vi "Main.vi"() -> ()   [LabVIEW 2020]
doc: "Use this template to build a simple state machine design pattern. Each state executes code and determines which state to transition to."
uses:
  controls/State.ctl
  controls/Data.ctl
  <vilib>/DAQmx/configure/timing.llb/DAQmx Timing (Sample Clock).vi
  <vilib>/DAQmx/create/channels.llb/DAQmx Create Channel (AI-Voltage-Basic).vi
  <vilib>/daqmxs/DAQmx sim.lvlib
  <vilib>/Waveform/WDTOps.llb/WDT Append Waveforms DBL.vi
  <vilib>/daqmxs/DAQmx Read sim (Analog Wfm 1Chan NSamp).vi
panel:
  in  "git pokus":bool
  in  "Init measurement":bool
  in  "stop":bool
  out "Waveform Graph":waveform(dbl)(graph)
  in  "Start Measurement":bool
  in  "rate":dbl=1000.0
  in  "physical channels 2":tag
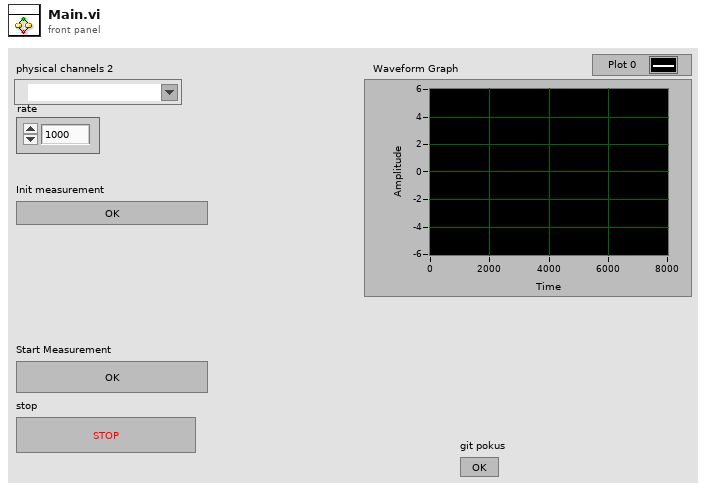
[diagram p1: front panel]
types:
  T1 = typedef "Data.ctl" = cluster{"Boolean ":bool, "String <Replace Me>":string, "Numeric <Replace Me>":dbl, "task out":refnum<k21>, "Waveform":waveform(dbl), "Numeric":i32}
  T2 = typedef "State.ctl" = enum16{"Initialize", "Wait for Event", "Run_measurement", "Exit", "Stop_measurement", "Read_measurement", "Init_measurement"}
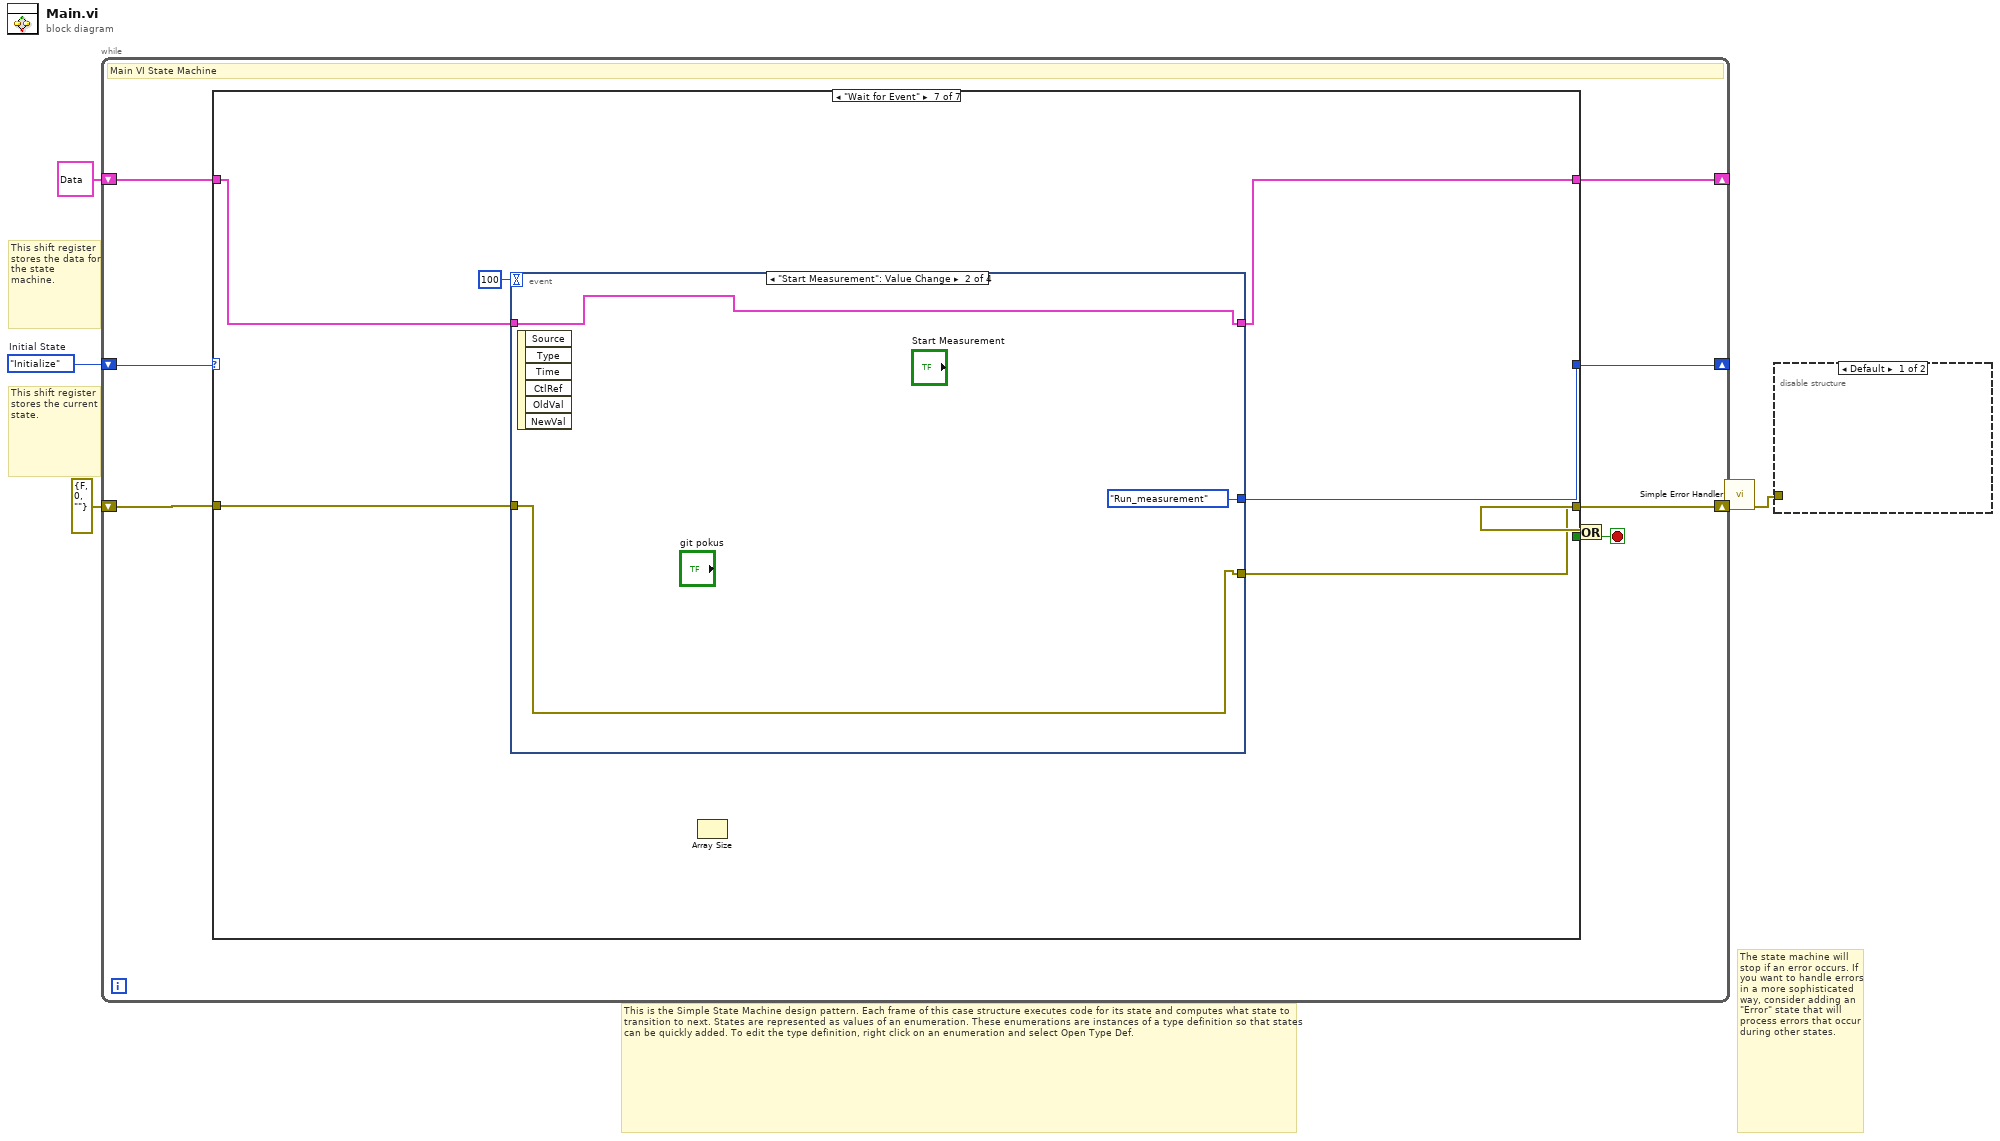
[diagram p0: block diagram]
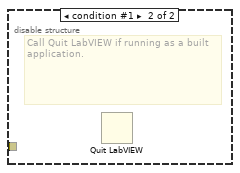
[diagram p2: hidden frame]
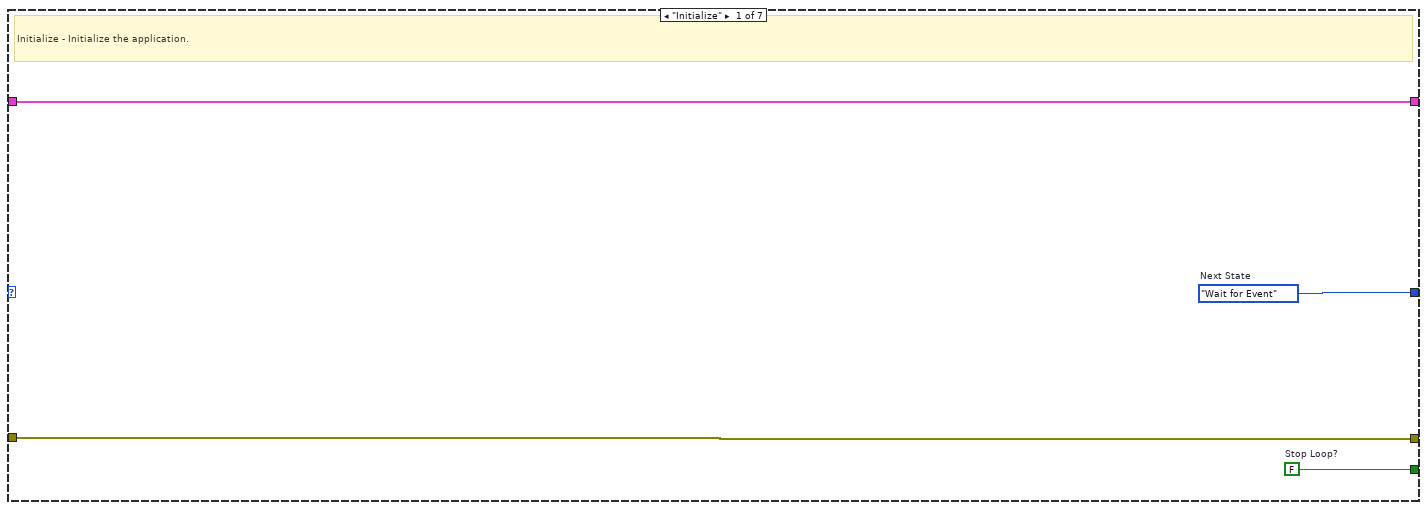
[diagram p3: hidden frame]
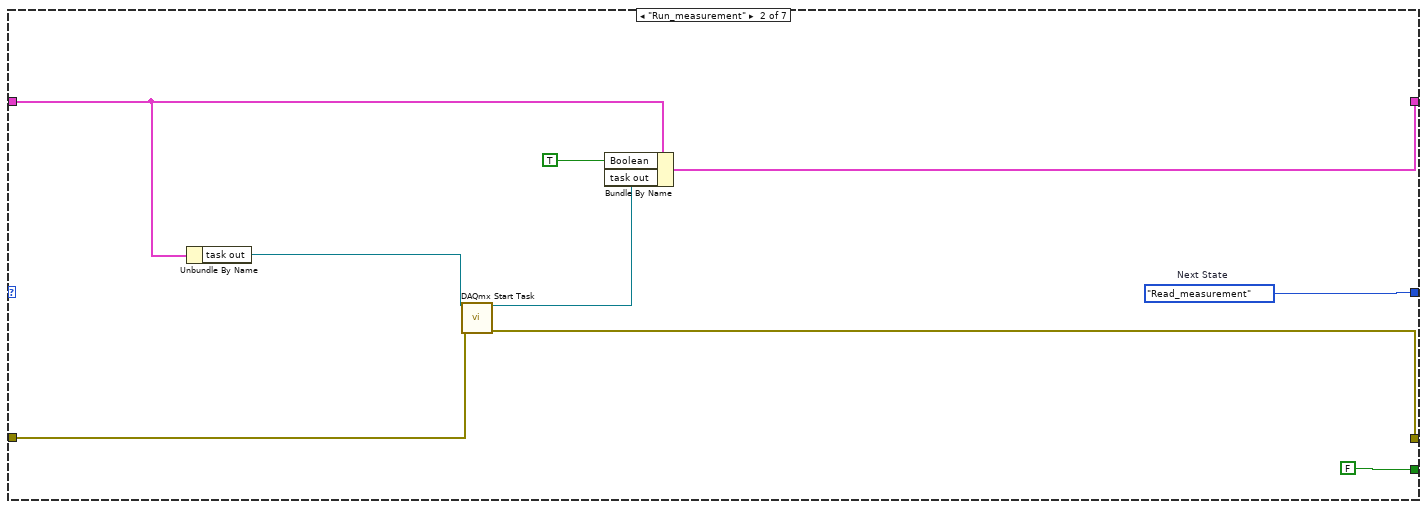
[diagram p4: hidden frame]
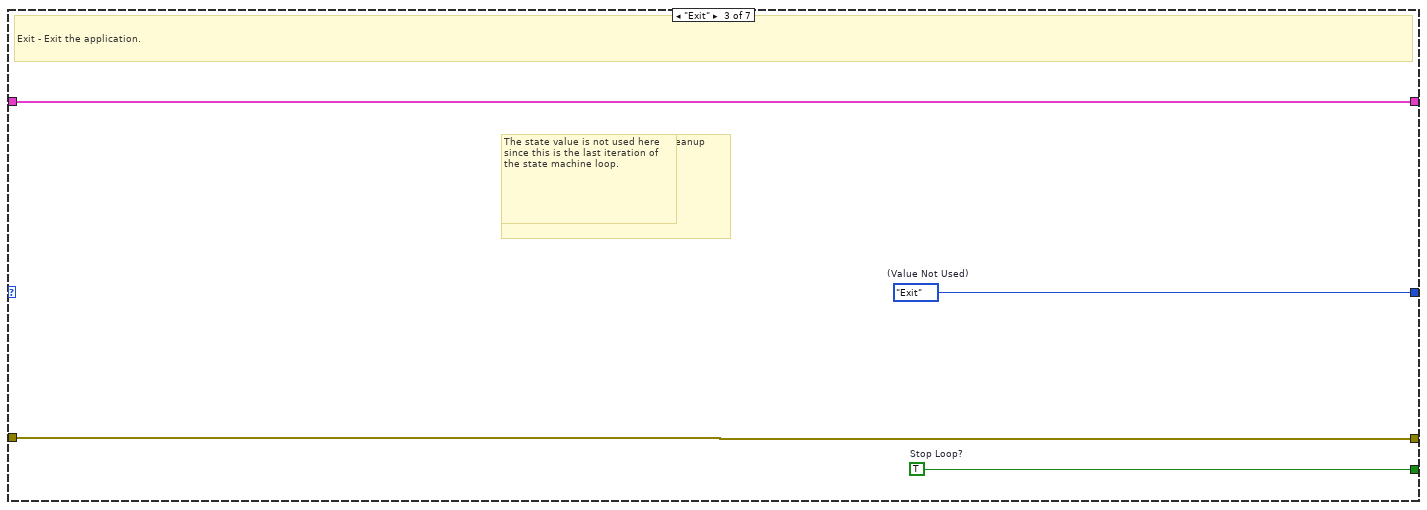
[diagram p5: hidden frame]
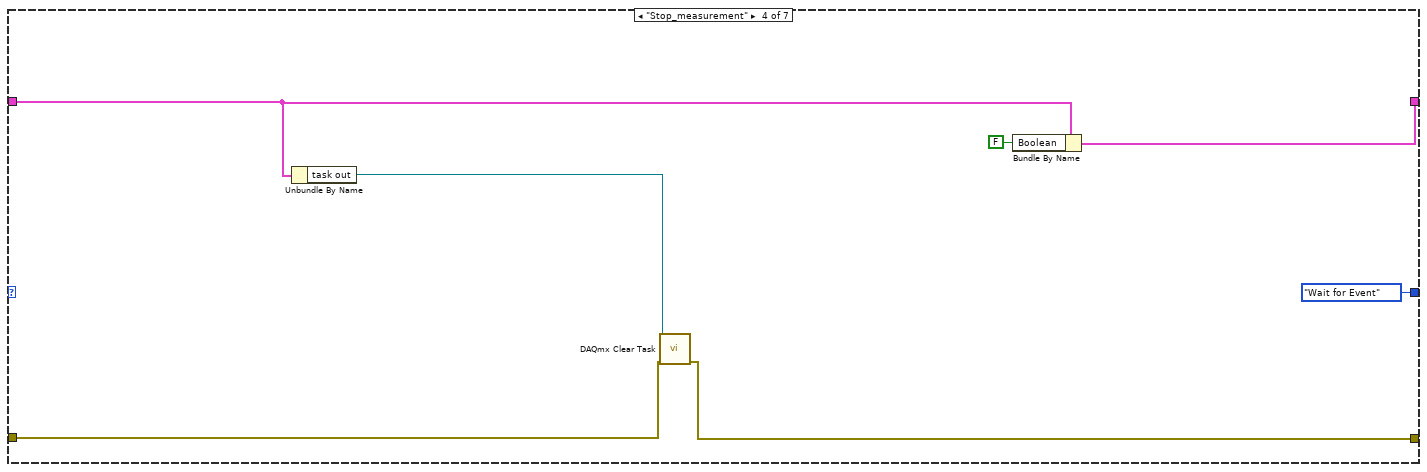
[diagram p6: hidden frame]
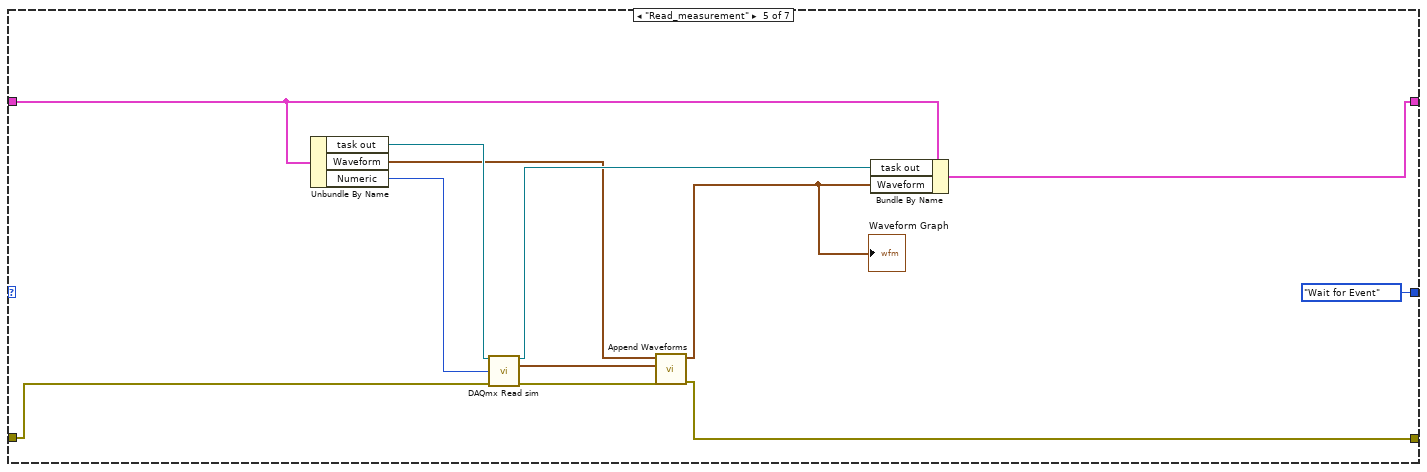
[diagram p7: hidden frame]
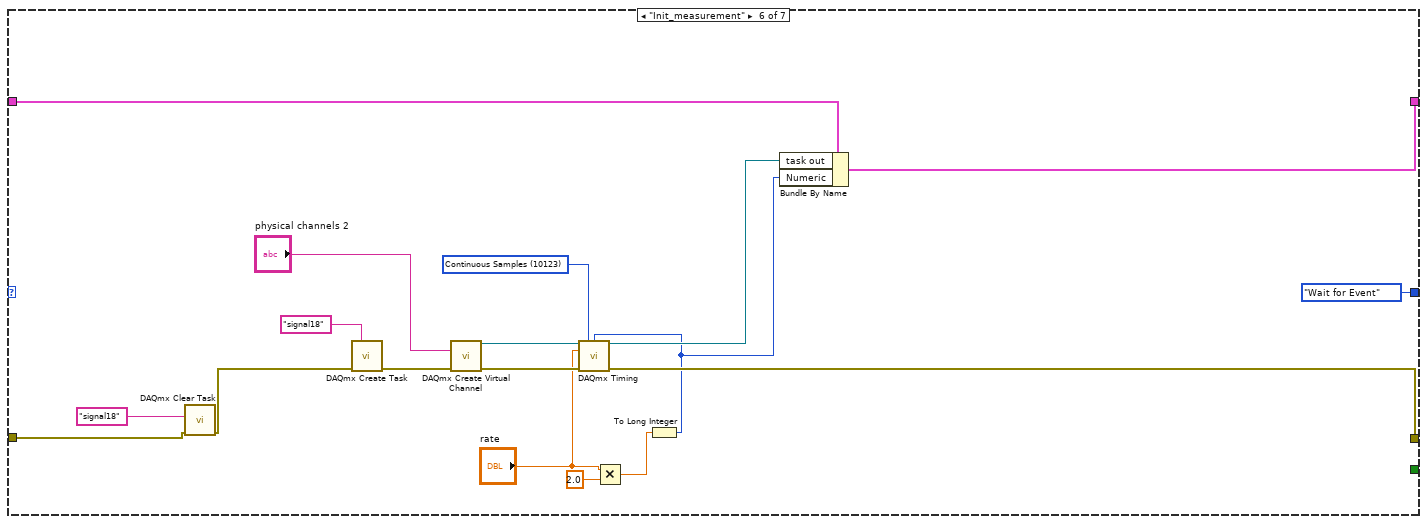
[diagram p8: hidden frame]
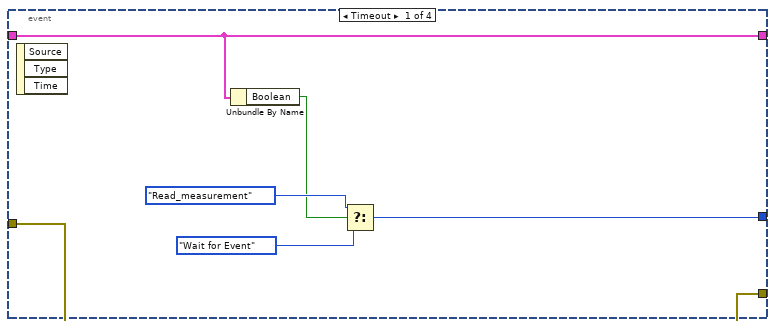
[diagram p9: hidden frame]
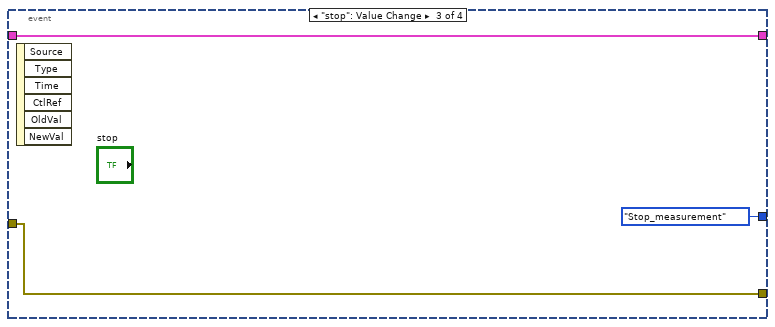
[diagram p10: hidden frame]
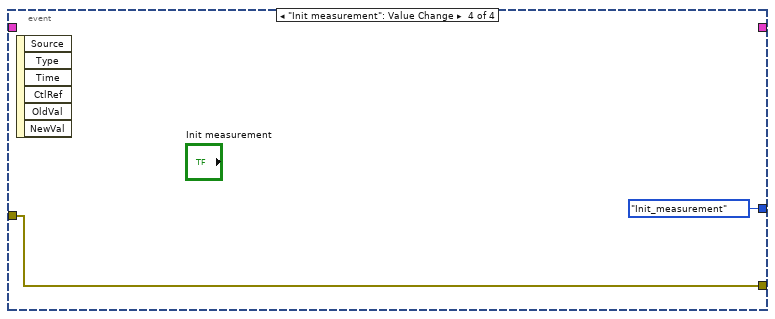
[diagram p11: hidden frame]
diagram:
  w5 = State."Initialize"  # Initial State
  # "The state machine will stop if an error occurs. If you want to handle errors in a more sophisticated way, consider adding an \"Error\" state that will process errors that occur during other states."
  # "This shift register stores the data for the state machine."
  # "This is the Simple State Machine design pattern. Each frame of this case structure executes code for its state and computes what state to transition to next. States are represented as values of an enumeration. These enumerations are instances of a type definition so that states can be quickly added. To edit the type definition, right click on an enumeration and select Open Type Def."
  # "This shift register stores the current state."
  n1 = while {
    shift-right: [w12] -> _
    shift-left: w5 -> [w13]
    shift-right: [w10] -> _
    shift-left: T1 {"Boolean "=FALSE, "String <Replace Me>"="", "Numeric <Replace Me>"=0.0, "task out"="", "Waveform"={"t0"=timestamp(0 s since 1904-01-01), "dt"=1.0, "Y"=[]}, "Numeric"=0} ("Data") -> [w11]
    shift-right: [w6] -> w2
    shift-left: errorcluster {"status"=FALSE, "code"=0, "source"=""} ("error constant") -> [w9]
    stop <- w7 stop-if-true
    # "Main VI State Machine"
    n2 = case shown="\"Wait for Event\"" w13 {
      tunnel: [w17 w25 w30 State."Wait for Event" ("(Value Not Used)") State."Wait for Event" ("(Value Not Used)") State."Wait for Event" ("(Value Not Used)") w72] -> w12
      tunnel: [w16 FALSE ("Stop Loop?") w28 _ _ _ _] -> w8
      tunnel: w11 -> [w14 w21 w29 w34 w47 w58 w69]
      tunnel: [w14 w20 w29 w33 w46 w57 w68] -> w10
      tunnel: w9 -> [w15 w24 w27 w36 w40 w59 w71]
      tunnel: [w15 w23 w27 w35 w39 w54 w70] -> w6
      frame "Initialize" {
        w16 = FALSE  # Stop Loop?
        w17 = State."Wait for Event"  # Next State
        # "Initialize - Initialize the application."
      }
      frame "Run_measurement" {
        w25 = State."Read_measurement"  # Next State
        n3 = Unbundle By Name(w21) -> ("task out"=w22:refnum<k21>)
        n4 = call <vilib>:"DAQmx Start Task.vi"("task/channels in"=w22, "error in"=w24) -> ("task out"=w19:refnum<k21>, "error out"=w23:errorcluster)  [unwired: 12 in]
        n5 = Bundle By Name(cluster=w21, "Boolean"=TRUE ("Boolean <Replace Me>"), "task out"=w19) -> (w20:T1)
      }
      frame "Exit" {
        w28 = TRUE  # Stop Loop?
        w30 = State."Exit"  # (Value Not Used)
        # "#CodeNeeded - Add any required cleanup code here."
        # "The state value is not used here since this is the last iteration of the state machine loop."
        # "Exit - Exit the application."
      }
      frame "Stop_measurement" {
        n6 = Unbundle By Name(w34) -> ("task out"=w37:refnum<k21>)
        n7 = call <vilib>:"DAQmx Clear Task.vi"("task in"=w37, "error in"=w36) -> ("error out"=w35:errorcluster)  [unwired: 13 in]
        n8 = Bundle By Name(cluster=w34, "Boolean"=FALSE) -> (w33:T1)
      }
      frame "Read_measurement" {
        n9 = Unbundle By Name(w47) -> ("task out"=w48:refnum<k21>, "Waveform"=w44:waveform(dbl), "Numeric"=w38:i32)
        n10 = call-poly <vilib>:"DAQmx Read sim.vi"("task/channels in"=w48, "number of samples per channel"=w38, "error in"=w40) -> ("task out"=w45:refnum<k21>, "data"=w43:waveform(dbl), "error out"=w41:errorcluster)  [unwired: 10 in]
        n11 = call-poly <vilib>:"Append Waveforms.vi"("error in (no error)"=w41, "waveform B"=w43, "waveform A"=w44) -> ("error out"=w39:errorcluster, "waveform out"=w42:waveform(dbl))  [unwired: 7 in]
        "Waveform Graph" <- w42
        n12 = Bundle By Name(cluster=w47, "task out"=w45, "Waveform"=w42) -> (w46:T1)
      }
      frame "Init_measurement" {
        w61 = 10123 items=["Finite Samples"=10178, "Continuous Samples"=10123, "Hardware Timed Single Point"=12522] ("sample mode")
        n13 = call <vilib>:"DAQmx Clear Task.vi"("task in"="signal18" ("new task name"), "error in"=w59) -> ("error out"=w60:errorcluster)  [unwired: 13 in]
        n14 = call <vilib>:"DAQmx Create Task.vi"("new task name"="signal18", "error in"=w60) -> ("error out"=w67:errorcluster)  [unwired: 12 in, 1 out]
        n15 = call-poly <vilib>:"DAQmx Create Virtual Channel.vi"("physical channels"="physical channels 2", "error in"=w67) -> ("task out"=w66:refnum<k21>, "error out"=w65:errorcluster)  [unwired: 12 in]
        n16 = Multiply(x="rate", y=2.0) -> (x*y=w51:dbl)
        n17 = To Long Integer(number=w51) -> (32bit integer=w50:i32)
        n18 = call-poly <vilib>:"DAQmx Timing.vi"("task/channels in"=w66, "sample mode"=w61, "samples per channel"=w50, "rate"="rate", "error in"=w65) -> ("task out"=w56:refnum<k21>, "error out"=w54:errorcluster)  [unwired: 9 in]
        n19 = Bundle By Name(cluster=w58, "task out"=w56, "Numeric"=w50) -> (w57:T1)
      }
      frame "Wait for Event" {
        n20 = event shown="[1] \"Start Measurement\": Value Change" {
          selector: _ -> [_ _ _ _]
          dyn-events: _ -> [_ _ _ _]
          timeout: 100 -> [_ _ _ _]
          tunnel: [w77 State."Run_measurement" ("(Value Not Used)") State."Stop_measurement" ("(Value Not Used)") State."Init_measurement" ("(Value Not Used)")] -> w72
          tunnel: w71 -> [w76 w82 w84 w86]
          tunnel: [w76 w82 w84 w86] -> w70
          tunnel: w69 -> [w74 w80 w83 _]
          tunnel: [w74 w80 w83 _] -> w68
          event Timeout {
            n21 = event-data() -> ()  [unwired: 1 in, 3 out]
            n22 = Unbundle By Name(w74) -> ("Boolean"=w75:bool)
            n23 = Select(t=State."Read_measurement" ("(Value Not Used)"), s=w75, f=State."Wait for Event" ("(Value Not Used)")) -> (s? t:f=w77:T2)
          }
          event "Start Measurement": Value Change {
            n24 = event-data() -> ()  [unwired: 1 in, 6 out]
          }
          event "stop": Value Change {
            n25 = event-data() -> ()  [unwired: 1 in, 6 out]
          }
          event "Init measurement": Value Change {
            n26 = event-data() -> ()  [unwired: 1 in, 6 out]
          }
        }
        n27 = Array Size() -> ()  [unwired: 1 in, 1 out]
      }
    }
    n28 = Or(x=w6, y=w8) -> (x .or. y?=w7:bool)
  }
  n29 = call <vilib>:"Simple Error Handler.vi"("error in (no error)"=w2) -> ("error out"=w1:errorcluster)  [unwired: 4 in, 4 out]
  n30 = disable-structure shown="Default" {
    disable-tunnel: w1 -> [_ _]
    frame condition #0 (active) {
    }
    frame condition #1 {
      # "Call Quit LabVIEW if running as a built application."
      n31 = Quit LabVIEW() -> ()  [unwired: 1 in]
    }
  }
